vi "Tag Memory.vi"(0 "Method":T5, 1 "Tags":string[](array[string]), 3 "Tag In":T2, 5 "Tag":string, 9 "Expected Type":T3, 11 "error in (no error)":errorcluster, 13 "Tag.Description":string) -> (4 "Index Out":i32, 6 "Description":string, 10 "Indices Out":i32[](array[numeric]), 12 "Group Indices Out":T4[](array[typedef]), 14 "Stored Tags":T1[](array[typedef]), 15 "error out":errorcluster)   [LabVIEW 2020, in "Current Value Table(Rebuild).lvlib"]
doc: "This VI stores the indices of every tag in the system, along with their type."
uses:
  Current Value Table(Rebuild).lvlib
  Tag Memory Methods.ctl
  Type Defs/Index Types.ctl
  Type Defs/Data Types.ctl
  Type Defs/Single Tag.ctl
  Type Defs/Tag in Memory.ctl
  ASCII String To Data.vi
  DataTypes/Double_ASCII String To Data.vi
  DataTypes/Array of String_ASCII String To Data.vi
  DataTypes/Array of Boolean_ASCII String To Data.vi
  DataTypes/Array of Single_ASCII String To Data.vi
  DataTypes/Array of Double_ASCII String To Data.vi
  DataTypes/Array of I8_ASCII String To Data.vi
  DataTypes/Array of I16_ASCII String To Data.vi
  DataTypes/Array of I32_ASCII String To Data.vi
  DataTypes/Array of I64_ASCII String To Data.vi
  DataTypes/Array of U64_ASCII String To Data.vi
  DataTypes/Array of U32_ASCII String To Data.vi
  DataTypes/Array of U16_ASCII String To Data.vi
  DataTypes/Array of U8_ASCII String To Data.vi
  DataTypes/Boolean_ASCII String To Data.vi
  DataTypes/String_ASCII String To Data.vi
  DataTypes/U8_ASCII String To Data.vi
  DataTypes/U16_ASCII String To Data.vi
  DataTypes/U32_ASCII String To Data.vi
  DataTypes/U64_ASCII String To Data.vi
  DataTypes/I8_ASCII String To Data.vi
  DataTypes/I16_ASCII String To Data.vi
  DataTypes/I32_ASCII String To Data.vi
  DataTypes/I64_ASCII String To Data.vi
  DataTypes/Single_ASCII String To Data.vi
  Errors/Scanned Value Error.vi
  Memory Block.vi
  DataTypes/Double_Memory Block.vi
  DataTypes/Array of String_Memory Block.vi
  DataTypes/Array of Boolean_Memory Block.vi
  DataTypes/Array of Single_Memory Block.vi
  DataTypes/Array of Double_Memory Block.vi
  DataTypes/Array of I8_Memory Block.vi
  DataTypes/Array of I16_Memory Block.vi
  DataTypes/Array of I32_Memory Block.vi
  DataTypes/Array of I64_Memory Block.vi
  DataTypes/Array of U64_Memory Block.vi
  DataTypes/Array of U32_Memory Block.vi
  DataTypes/Array of U16_Memory Block.vi
  DataTypes/Array of U8_Memory Block.vi
  DataTypes/Boolean_Memory Block.vi
  DataTypes/String_Memory Block.vi
  DataTypes/U8_Memory Block.vi
  DataTypes/U16_Memory Block.vi
  DataTypes/U32_Memory Block.vi
  DataTypes/U64_Memory Block.vi
  DataTypes/I8_Memory Block.vi
  DataTypes/I16_Memory Block.vi
  DataTypes/I32_Memory Block.vi
  DataTypes/I64_Memory Block.vi
  DataTypes/Single_Memory Block.vi
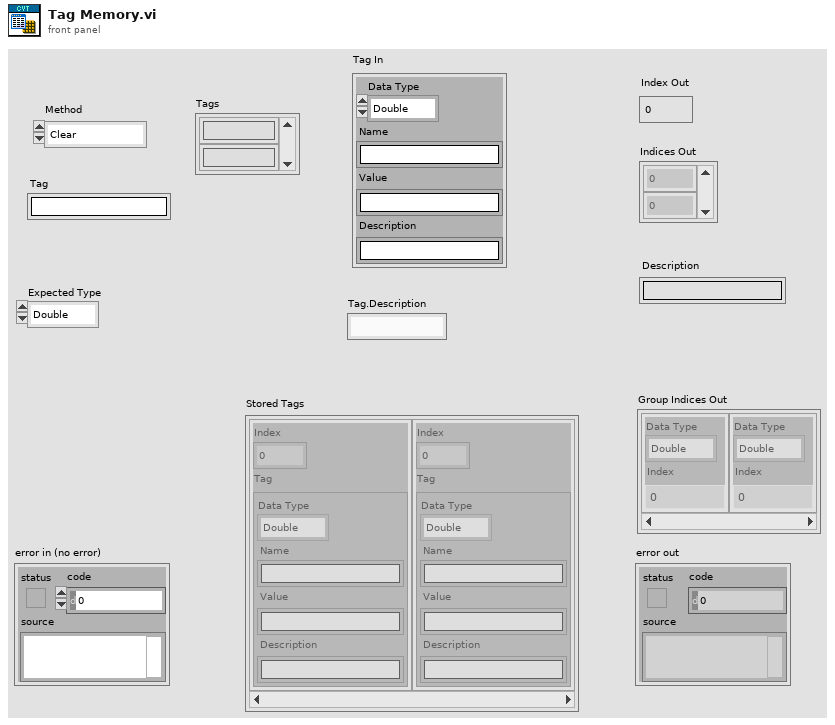
[diagram p1: front panel]
types:
  T1 = typedef "Current Value Table(Rebuild).lvlib/Tag in Memory.ctl" = cluster{"Index":i32, "Tag":T2}
  T2 = typedef "Current Value Table(Rebuild).lvlib/Single Tag.ctl" = cluster{"Data Type":T3, "Name":string, "Value":string, "Description":string}
  T3 = typedef "Current Value Table(Rebuild).lvlib/Data Types.ctl" = enum16{"Double", "Single", "I64", "I32", "I16", "I8", "U64", "U32", "U16", "U8", "String", "Boolean", "Array of U8", "Array of U16", "Array of U32", "Array of U64", "Array of I64", "Array of I32", "Array of I16", "Array of I8", "Array of Double", "Array of Single", "Array of Boolean", "Array of String"}
  T4 = typedef "Current Value Table(Rebuild).lvlib/Index Types.ctl" = cluster{"Data Type":T3, "Index":i32}
  T5 = typedef "Current Value Table(Rebuild).lvlib/Tag Memory Methods.ctl" = enum16{"Clear", "Read Tag Index", "Read Tag Indices", "Generate Group", "Add Tag", "Overwrite Tag", "Read Description", "Get Stored Tags", "Write Description"}
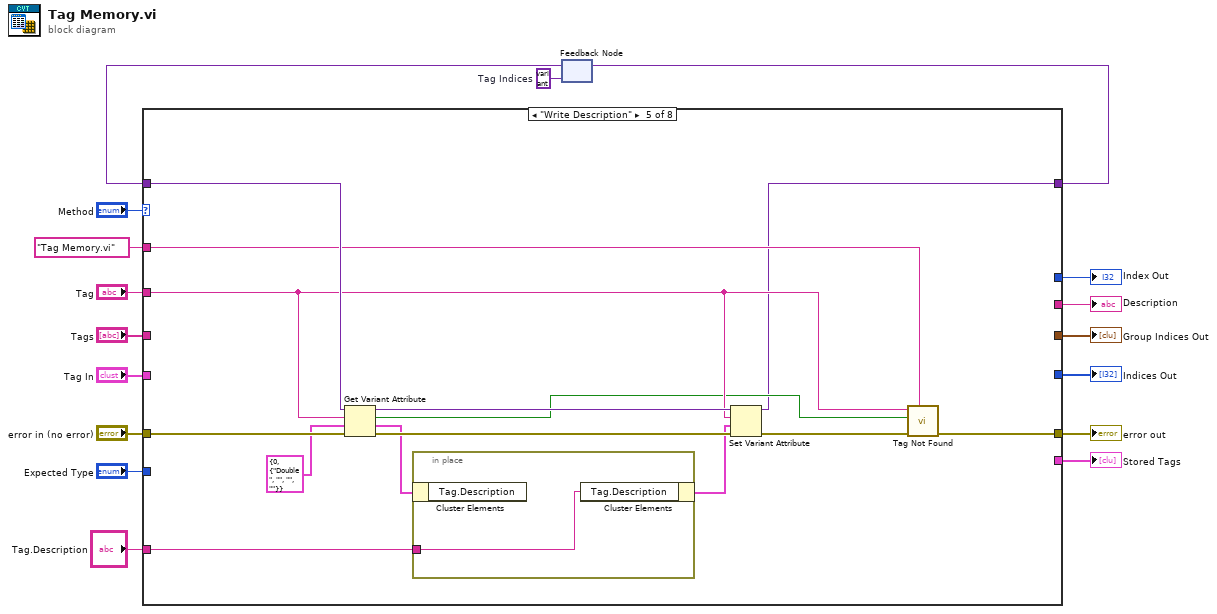
[diagram p0: block diagram]
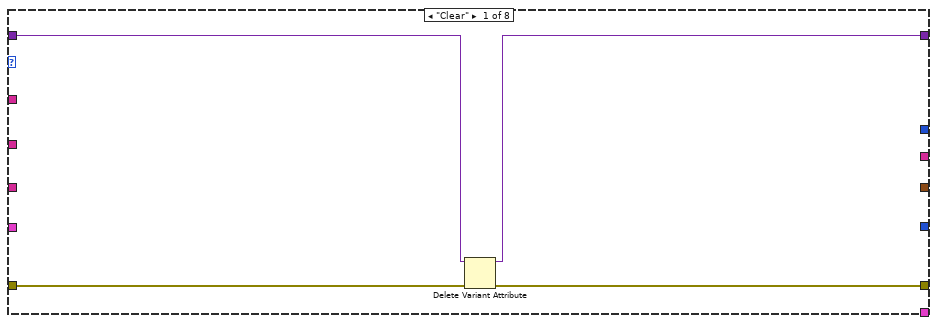
[diagram p2: hidden frame]
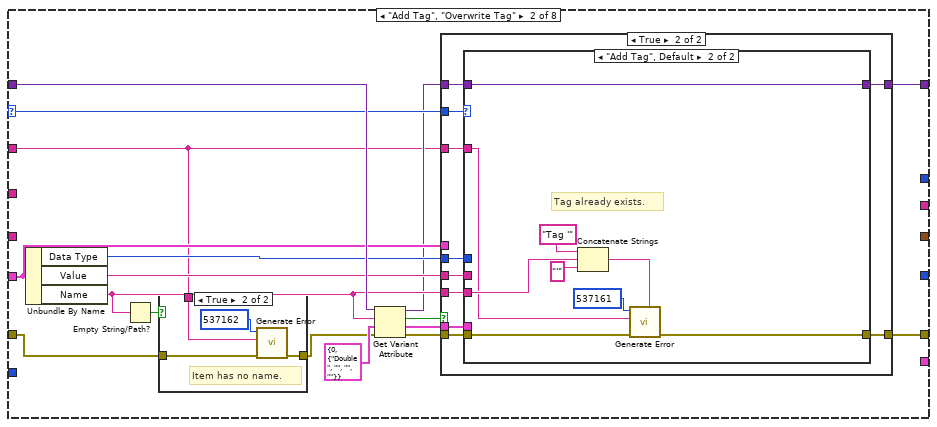
[diagram p3: hidden frame]
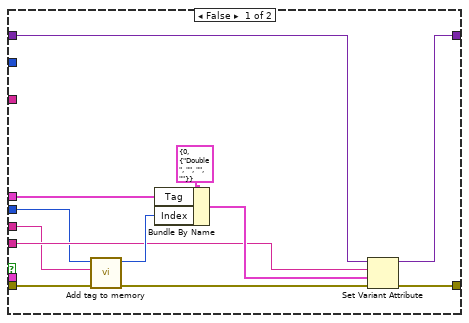
[diagram p5: hidden frame]
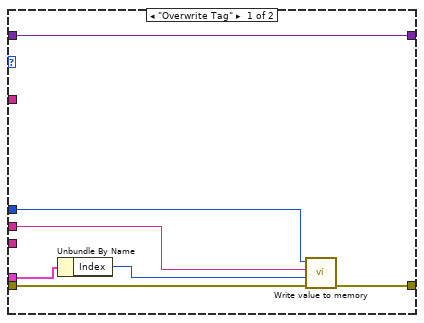
[diagram p6: hidden frame]
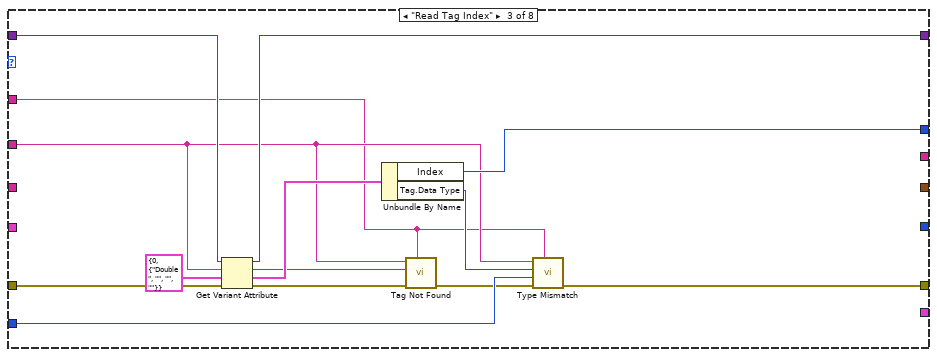
[diagram p7: hidden frame]
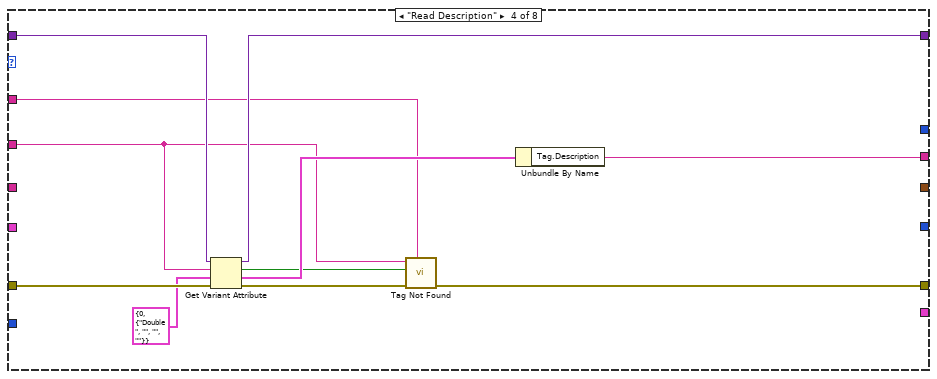
[diagram p8: hidden frame]
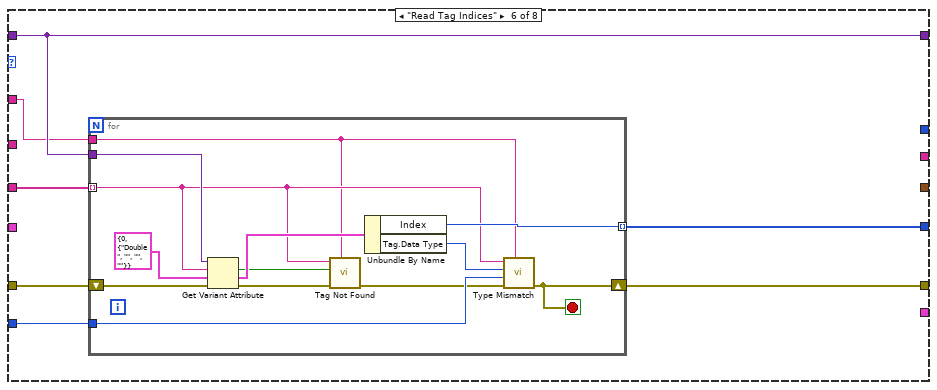
[diagram p9: hidden frame]
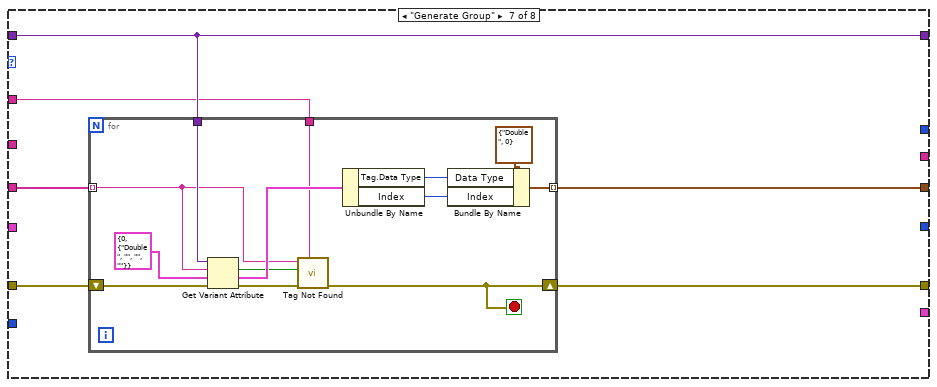
[diagram p10: hidden frame]
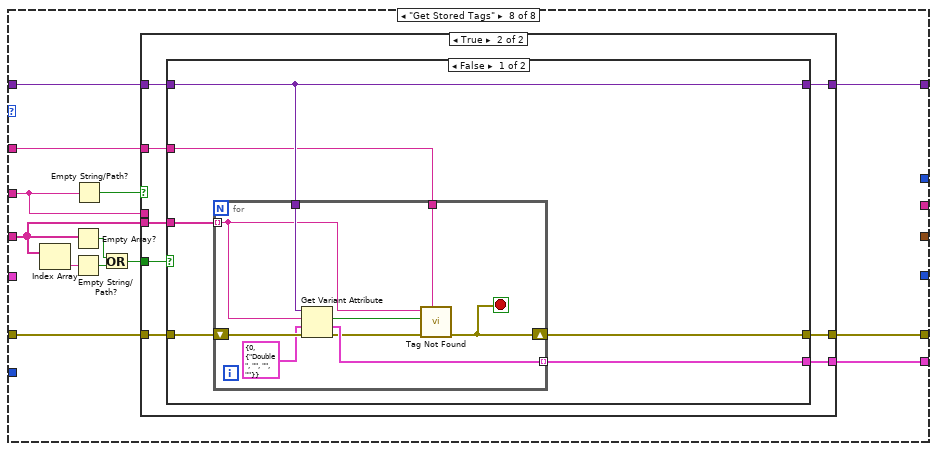
[diagram p11: hidden frame]
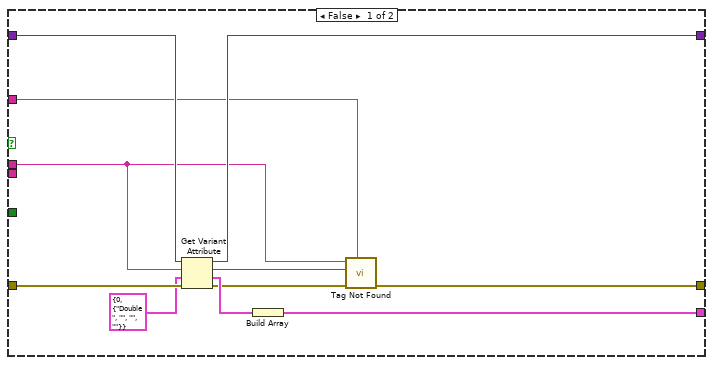
[diagram p12: hidden frame]
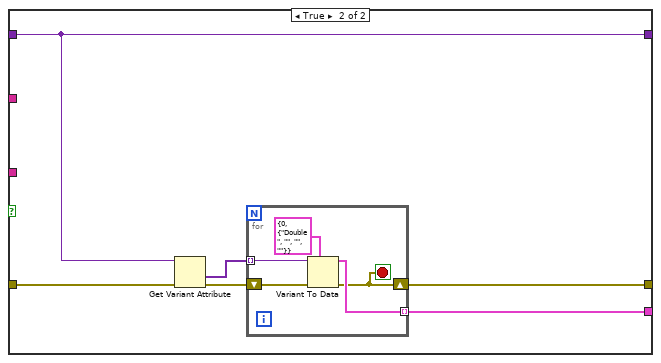
[diagram p13: hidden frame]
diagram:
  w17 = variant  # Tag Indices
  n1 = feedback #1(w17) -> (w15:variant)
  n2 = case shown="\"Write Description\"" "Method" {
    selector: "Method" -> [_ w29 _ _ _ _ _ _]
    tunnel: w15 -> [w19 w38 w94 w105 w118 w125 w144 w168]
    tunnel: [w18 w26 w93 w104 w107 w125 w144 w167] -> w14
    tunnel: "Tag In" -> [_ w36 _ _ _ _ _ _]
    tunnel: "error in (no error)" -> [w21 w24 w95 w106 w119 w127 w146 w170]
    tunnel: [w20 w27 w89 w99 w116 w126 w145 w166] -> w11
    tunnel: "Tags" -> [_ _ _ _ _ w124 w143 w161]
    tunnel: [_ _ _ _ _ _ w142 _] -> w9
    tunnel: "Tag" -> [_ _ w84 w98 w110 _ _ w169]
    tunnel: "Expected Type" -> [_ _ w87 _ _ w123 _ _]
    tunnel: [_ _ w90 _ _ _ _ _] -> w6
    tunnel: [_ _ _ w101 _ _ _ _] -> w5
    tunnel: [_ _ _ _ _ _ _ w165] -> w4
    tunnel: [_ _ _ _ _ w122 _ _] -> w3
    tunnel: "Tag Memory.vi" ("caller name") -> [_ w22 w82 w96 w115 w121 w141 w160]
    tunnel: "Tag.Description" -> [_ _ _ _ w111 _ _ _]
    frame "Clear" {
      n3 = Delete Variant Attribute(4:w21, 7:w19) -> (0:w20:errorcluster, 3:w18:variant)  [unwired: 1 in, 1 out]
    }
    frame "Add Tag", "Overwrite Tag" {
      n4 = Unbundle By Name(w36) -> ("Data Type"=w34:T3, "Value"=w33:string, "Name"=w35:string)
      n5 = Empty String/Path?(string/path=w35) -> (empty?=w25:bool)
      n6 = case shown="True" w25 {
        tunnel: w24 -> [w39 w42]
        tunnel: [w39 w41] -> w23
        tunnel: w22 -> [_ w40]
        frame False {
        }
        frame True {
          # "Item has no name."
          n7 = call "Generate Error.vi"("error in"=w42, "caller name"=w40, "code"=537162) -> ("error out"=w41:errorcluster)  [unwired: 8 in]
        }
      }
      n8 = Get Variant Attribute(Variant=w38, name=w35, default value (empty Variant)=T1 {"Index"=0, "Tag"={"Data Type"=enum."Double", "Name"="", "Value"="", "Description"=""}} ("Tag"), error in=w23) -> (duplicate Variant=w28:variant, found=w31:bool, value=w30:T1, error out=w37:errorcluster)
      n9 = case shown="True" w31 {
        tunnel: w37 -> [w50 w64]
        tunnel: w36 -> [w48 _]
        tunnel: w35 -> [w47 w61]
        tunnel: [w55 w63] -> w27
        tunnel: w34 -> [w45 w60]
        tunnel: w33 -> [w46 w59]
        tunnel: w30 -> [_ w62]
        tunnel: w29 -> [_ w65]
        tunnel: w28 -> [w54 w58]
        tunnel: [w53 w57] -> w26
        tunnel: w22 -> [_ w56]
        frame False {
          n10 = call "Add tag to memory.vi"("error in (no error)"=w50, "Value"=w46, "Data Type"=w45) -> ("error out"=w44:errorcluster, "Index"=w51:i32)  [unwired: 7 in]
          n11 = Bundle By Name(cluster=T1 {"Index"=0, "Tag"={"Data Type"=enum."Double", "Name"="", "Value"="", "Description"=""}} ("Tag"), "Tag"=w48, "Index"=w51) -> (w49:T1)
          n12 = Set Variant Attribute(Variant=w54, name=w47, value=w49, error in=w44) -> (Variant out=w53:variant, error out=w55:errorcluster)  [unwired: 1 out]
        }
        frame True {
          n13 = case shown="\"Add Tag\", Default" w65 {
            tunnel: w64 -> [w72 w75]
            tunnel: [w71 w74] -> w63
            tunnel: w62 -> [w67 _]
            tunnel: w61 -> [_ w77]
            tunnel: w60 -> [w70 _]
            tunnel: w59 -> [w69 _]
            tunnel: w58 -> [w66 w81]
            tunnel: [w66 w81] -> w57
            tunnel: w56 -> [_ w73]
            frame "Overwrite Tag" {
              n14 = Unbundle By Name(w67) -> ("Index"=w68:i32)
              n15 = call "Write value to memory.vi"("error in (no error)"=w72, "Index"=w68, "Value"=w69, "Data Type"=w70) -> ("error out"=w71:errorcluster)  [unwired: 7 in]
            }
            frame "Add Tag", Default {
              # "Tag already exists."
              n16 = Concatenate Strings("Tag '" ("string"), w77, "'" ("string")) -> (w76:string)
              n17 = call "Generate Error.vi"("<append> (\"\")"=w76, "error in"=w75, "caller name"=w73, "code"=537161) -> ("error out"=w74:errorcluster)  [unwired: 7 in]
            }
          }
        }
      }
    }
    frame "Read Tag Index" {
      n18 = Get Variant Attribute(Variant=w94, name=w84, default value (empty Variant)=T1 {"Index"=0, "Tag"={"Data Type"=enum."Double", "Name"="", "Value"="", "Description"=""}} ("Tag"), error in=w95) -> (duplicate Variant=w93:variant, found=w83:bool, value=w91:T1, error out=w86:errorcluster)
      n19 = Unbundle By Name(w91) -> ("Index"=w90:i32, "Tag.Data Type"=w88:T3)
      n20 = call "Tag Not Found.vi"("caller name"=w82, "error in (no error)"=w86, "found?"=w83, "Tag Name"=w84) -> ("error out"=w85:errorcluster)  [unwired: 7 in]
      n21 = call "Type Mismatch.vi"("caller name"=w82, "error in (no error)"=w85, "Data Type Requested"=w87, "True Type"=w88, "Tag"=w84) -> ("error out"=w89:errorcluster)  [unwired: 6 in]
    }
    frame "Read Description" {
      n22 = Get Variant Attribute(Variant=w105, name=w98, default value (empty Variant)=T1 {"Index"=0, "Tag"={"Data Type"=enum."Double", "Name"="", "Value"="", "Description"=""}} ("Tag"), error in=w106) -> (duplicate Variant=w104:variant, found=w97:bool, value=w102:T1, error out=w100:errorcluster)
      n23 = call "Tag Not Found.vi"("caller name"=w96, "error in (no error)"=w100, "found?"=w97, "Tag Name"=w98) -> ("error out"=w99:errorcluster)  [unwired: 7 in]
      n24 = Unbundle By Name(w102) -> ("Tag.Description"=w101:string)
    }
    frame "Write Description" {
      n25 = Get Variant Attribute(Variant=w118, name=w110, default value (empty Variant)=T1 {"Index"=0, "Tag"={"Data Type"=enum."Double", "Name"="", "Value"="", "Description"=""}} ("Tag"), error in=w119) -> (duplicate Variant=w113:variant, found=w108:bool, value=w112:T1, error out=w114:errorcluster)
      n26 = in-place {
        in-place-border: w111 -> [w120]
        n27 = in-place-cluster #2(w112) -> ()  [unwired: 1 out]
        n28 = in-place-cluster #2("Tag.Description"=w120) -> (w109:T1)
      }
      n29 = Set Variant Attribute(Variant=w113, name=w110, value=w109, error in=w114) -> (Variant out=w107:variant)  [unwired: 2 out]
      n30 = call "Tag Not Found.vi"("caller name"=w115, "error in (no error)"=w114, "found?"=w108, "Tag Name"=w110) -> ("error out"=w116:errorcluster)  [unwired: 7 in]
    }
    frame "Read Tag Indices" {
      n31 = for {
        shift-right: [w136] -> w126
        shift-left: w127 -> [w140]
        tunnel: w125 -> [w138]
        tunnel: w124 -> [w132] mode=indexing
        tunnel: w123 -> [w135]
        tunnel: [w133] -> w122 mode=indexing
        tunnel: w121 -> [w128]
        stop <- w136 stop-if-true
        n32 = Get Variant Attribute(Variant=w138, name=w132, default value (empty Variant)=T1 {"Index"=0, "Tag"={"Data Type"=enum."Double", "Name"="", "Value"="", "Description"=""}} ("Tag"), error in=w140) -> (found=w131:bool, value=w137:T1, error out=w130:errorcluster)  [unwired: 1 out]
        n33 = call "Tag Not Found.vi"("caller name"=w128, "error in (no error)"=w130, "found?"=w131, "Tag Name"=w132) -> ("error out"=w129:errorcluster)  [unwired: 7 in]
        n34 = Unbundle By Name(w137) -> ("Index"=w133:i32, "Tag.Data Type"=w134:T3)
        n35 = call "Type Mismatch.vi"("caller name"=w128, "error in (no error)"=w129, "Data Type Requested"=w135, "True Type"=w134, "Tag"=w132) -> ("error out"=w136:errorcluster)  [unwired: 6 in]
      }
    }
    frame "Generate Group" {
      n36 = for {
        shift-right: [w150] -> w145
        shift-left: w146 -> [w159]
        tunnel: w144 -> [w157]
        tunnel: w143 -> [w148] mode=indexing
        tunnel: [w155] -> w142 mode=indexing
        tunnel: w141 -> [w147]
        stop <- w150 stop-if-true
        n37 = Get Variant Attribute(Variant=w157, name=w148, default value (empty Variant)=T1 {"Index"=0, "Tag"={"Data Type"=enum."Double", "Name"="", "Value"="", "Description"=""}} ("Tag"), error in=w159) -> (found=w149:bool, value=w154:T1, error out=w151:errorcluster)  [unwired: 1 out]
        n38 = call "Tag Not Found.vi"("caller name"=w147, "error in (no error)"=w151, "found?"=w149, "Tag Name"=w148) -> ("error out"=w150:errorcluster)  [unwired: 7 in]
        n39 = Unbundle By Name(w154) -> ("Tag.Data Type"=w152:T3, "Index"=w153:i32)
        n40 = Bundle By Name(cluster=T4 {"Data Type"=enum."Double", "Index"=0} ("Index Type"), "Data Type"=w152, "Index"=w153) -> (w155:T4)
      }
    }
    frame "Get Stored Tags" {
      n41 = Index Array(array=w161) -> (element=w172:string)  [unwired: 1 in]
      n42 = Empty Array?(array=w161) -> (empty?=w163:bool)
      n43 = Empty String/Path?(string/path=w172) -> (empty?=w164:bool)
      n44 = Empty String/Path?(string/path=w169) -> (empty?=w171:bool)
      n45 = Or(x=w163, y=w164) -> (x .or. y?=w162:bool)
      n46 = case shown="True" w171 {
        tunnel: w170 -> [w183 w191]
        tunnel: w169 -> [w174 _]
        tunnel: w168 -> [w182 w188]
        tunnel: [w181 w187] -> w167
        tunnel: [w176 w190] -> w166
        tunnel: [w178 w186] -> w165
        tunnel: w162 -> [_ w189]
        tunnel: w161 -> [_ w185]
        tunnel: w160 -> [w173 w184]
        frame False {
          n47 = Get Variant Attribute(Variant=w182, name=w174, default value (empty Variant)=T1 {"Index"=0, "Tag"={"Data Type"=enum."Double", "Name"="", "Value"="", "Description"=""}} ("Tag"), error in=w183) -> (duplicate Variant=w181:variant, found=w175:bool, value=w179:T1, error out=w177:errorcluster)
          n48 = Build Array(w179) -> (w178:T1[])
          n49 = call "Tag Not Found.vi"("caller name"=w173, "error in (no error)"=w177, "found?"=w175, "Tag Name"=w174) -> ("error out"=w176:errorcluster)  [unwired: 7 in]
        }
        frame True {
          n50 = case shown="False" w189 {
            tunnel: w191 -> [w197 w212]
            tunnel: [w196 w209] -> w190
            tunnel: w188 -> [w194 w211]
            tunnel: [w194 w211] -> w187
            tunnel: [w193 w207] -> w186
            tunnel: w185 -> [w195 _]
            tunnel: w184 -> [w192 _]
            frame False {
              n51 = for {
                shift-right: [w201] -> w196
                shift-left: w197 -> [w206]
                tunnel: w195 -> [w199] mode=indexing
                tunnel: w194 -> [w204]
                tunnel: [w203] -> w193 mode=indexing
                tunnel: w192 -> [w198]
                stop <- w201 stop-if-true
                n52 = Get Variant Attribute(Variant=w204, name=w199, default value (empty Variant)=T1 {"Index"=0, "Tag"={"Data Type"=enum."Double", "Name"="", "Value"="", "Description"=""}} ("Tag"), error in=w206) -> (found=w200:bool, value=w203:T1, error out=w202:errorcluster)  [unwired: 1 out]
                n53 = call "Tag Not Found.vi"("caller name"=w198, "error in (no error)"=w202, "found?"=w200, "Tag Name"=w199) -> ("error out"=w201:errorcluster)  [unwired: 7 in]
              }
            }
            frame True {
              n54 = Get Variant Attribute(Variant=w211, error in=w212) -> (values=w208:variant[], error out=w210:errorcluster)  [unwired: 2 in, 2 out]
              n55 = for {
                shift-right: [w213] -> w209
                shift-left: w210 -> [w217]
                tunnel: w208 -> [w215] mode=indexing
                tunnel: [w214] -> w207 mode=indexing
                stop <- w213 stop-if-true
                n56 = Variant To Data(error in=w217, type=T1 {"Index"=0, "Tag"={"Data Type"=enum."Double", "Name"="", "Value"="", "Description"=""}} ("Tag"), Variant=w215) -> (data=w214:T1, error out=w213:errorcluster)
              }
            }
          }
        }
      }
    }
  }
  "error out" <- w11
  "Group Indices Out" <- w9
  "Index Out" <- w6
  "Description" <- w5
  "Stored Tags" <- w4
  "Indices Out" <- w3
  n57 = feedback-in #1(w14) -> ()
